vi "AngleStats_AngleAdd_CallbackHelp.vi"(9 "B":T1, 10 "A":T1, 11 "ExtraPassedData":variant) -> (0 "Error":bool, 3 "Result":T1)   [LabVIEW 2019, in "Trajectory_Library.lvlib"]
doc: "Returns a function that adds two vectors while normalizing the resulting value in the selected row as an angle. The calling parameters for this function adhere to to those required to be called as F or H functions.\n \n\nInputs:\n - ExtraPassedData -- Variant containing extra data passed to the function. For this instance the data contains.\n -- integer -- row -- The row containing angles to be normalized.\n - A -- A matrix\n - B -- B matrix\n\nOutputs:\n - Result -- Function returning of two vectors with angle at the given index normalized.\n - Error -- If TRUE, an error has occured."
uses:
  Trajectory_Library.lvlib
  <vilib>/Analysis/Matrix/Datatypes/RealMatrix.ctl
  <vilib>/Analysis/Matrix/NI_Matrix.lvlib
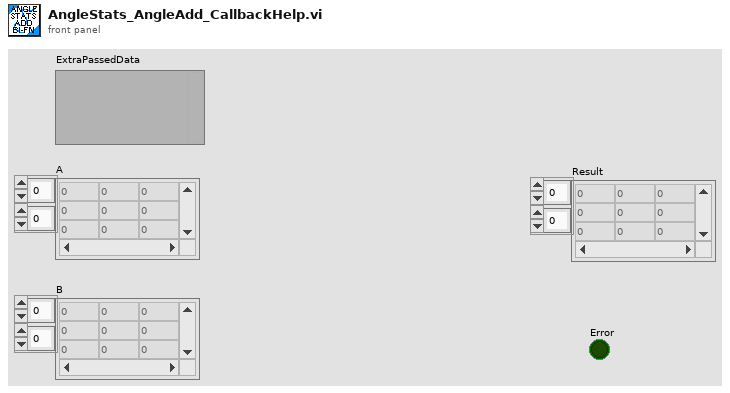
[diagram p1: front panel]
types:
  T1 = typedef "NI_Matrix.lvlib/RealMatrix.ctl" = dbl[][]
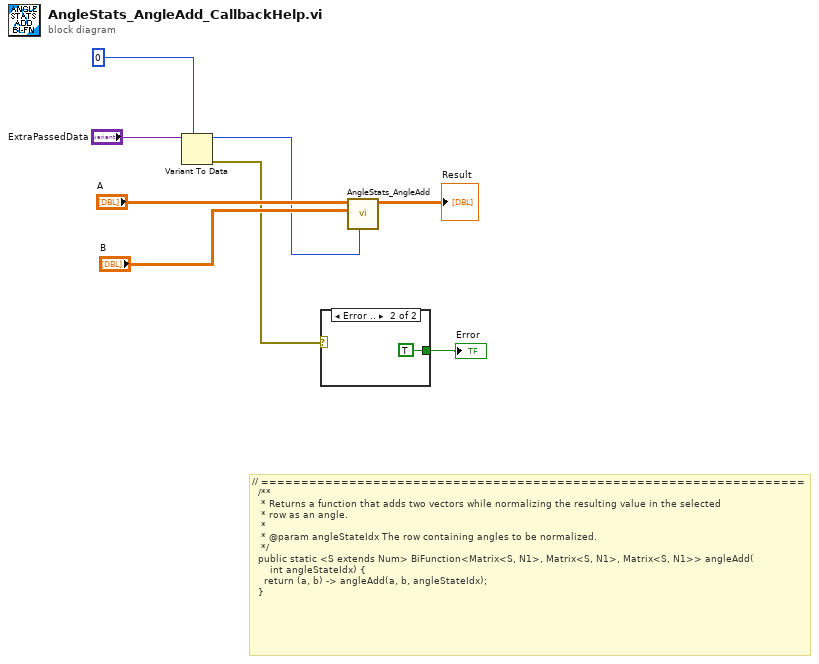
[diagram p0: block diagram]
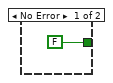
[diagram p2: hidden frame]
diagram:
  # "// ====================================================================\n  /**\n   * Returns a function that adds two vectors while normalizing the resulting value in the selected\n   * row as an angle.\n   *\n   * @param angleStateIdx The row containing angles to be normalized.\n   */\n  public static <S extends Num> BiFunction<Matrix<S, N1>, Matrix<S, N1>, Matrix<S, N1>> angleAdd(\n      int angleStateIdx) {\n    return (a, b) -> angleAdd(a, b, angleStateIdx);\n  }"
  n1 = Variant To Data(type=0, Variant="ExtraPassedData") -> (data=w4:i32, error out=w2:errorcluster)  [unwired: 1 in]
  n2 = case shown="Error .." w2 {
    tunnel: [FALSE TRUE] -> w1
    frame No Error {
    }
    frame Error {
    }
  }
  "Error" <- w1
  n3 = call "AngleStats_AngleAdd.vi"("Row"=w4, "B"="B", "A"="A") -> ("Result"=→"Result":T1)  [unwired: 8 in]
